vi "StartUp Sequence Open Loop Rev 1.55.vi"() -> ()   [LabVIEW 2017]
panel:
  out "Requested RPM":i32
  out "Waveform Chart":cluster{i32, i32}(graph)
  in  "Set RPM":string
  out "Pump Value 2":string
  in  "Soft Shut Off":bool
  out "Pump Value 1":string
  in  "Send RPM":bool
  in  "Send Command":bool
  in  "Custom Command":string
  out "Startup Success":bool
  in  "Output File":path
  in  "Shut Off":bool
  out "ECU COM Port Out":refnum<visa-resource-name>
  out "Throttle Position":string
  out "Turbine RPM":string
  out "Turbine Temp":string
  out "Error Out":errorcluster
  in  "Error In":errorcluster
  in  "ECU COM Port":refnum<visa-resource-name>
  out "Turbine State":string
  in  "Strt Sqnc":bool
  # "Note: save to a .csv file"
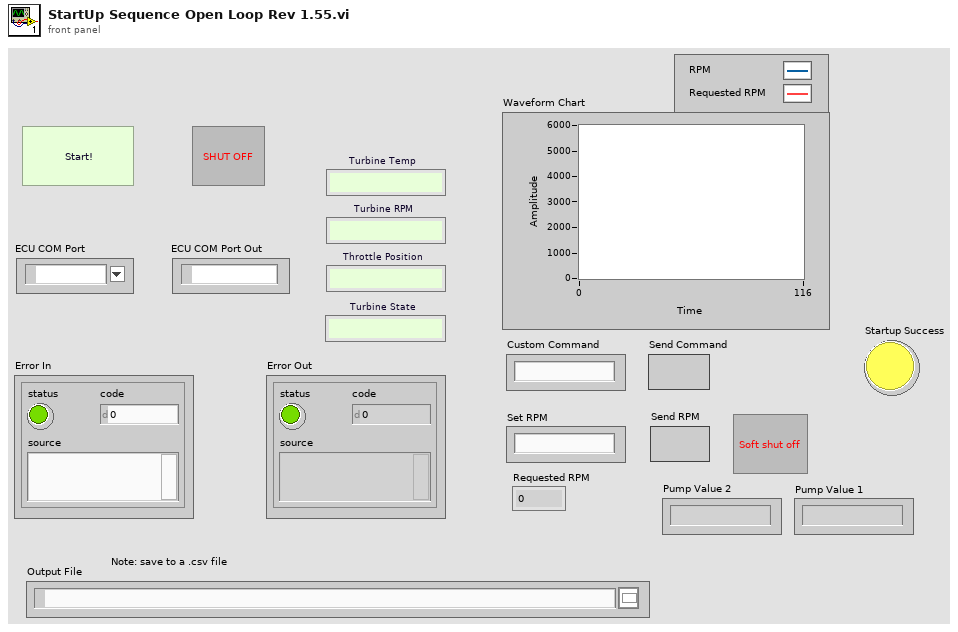
[diagram p1: front panel]
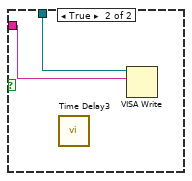
[diagram p3: hidden frame]
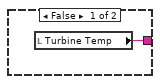
[diagram p4: hidden frame]
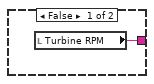
[diagram p5: hidden frame]
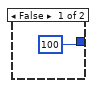
[diagram p7: hidden frame]
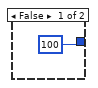
[diagram p8: hidden frame]
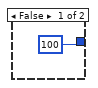
[diagram p9: hidden frame]
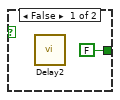
[diagram p11: hidden frame]
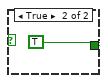
[diagram p12: hidden frame]
diagram:
  w27 = 21 ("Pulse Width")
  w28 = 160 ("Voltage")
  w33 = 16 ("Pulse Width")
  w34 = 160 ("Voltage")
  w24 = 255 ("y")
  w25 = 80 ("y")
  # "Disengage Starter Motor"
  # "Starter Motor 55%"
  # "Start button is inside a while loop that doesn't progess until True"
  # "Fuel Pump Mode 2"
  # "GlowPlugOff"
  # "Start Up\nFuelPumpMode 1"
  # "BurnerValveIgnitionPercent"
  # "If False, each Case structure is set\nto an arbitrary Delay time of 0.2 s"
  # "Each Stage is inside a while loop so that \nthe sequence doesn't progress until True"
  n1 = call "Initialize Com Port.vi"("Error In"="Error In", "ECU COM Port"="ECU COM Port") -> ("Error Out"=w47:errorcluster, "ECU COM Port Out"=w46:refnum<visa-resource-name>)  [unwired: 8 in]
  n2 = while {
    tunnel: w47 -> [w99]
    tunnel: [w99] -> w45
    stop <- "Strt Sqnc" stop-if-true
  }
  n3 = call "Initialize Output File.vi"("error in (no error)"=w45, "File Path Control"="Output File") -> ("error out"=w23:errorcluster)  [unwired: 9 in]
  n4 = flat-sequence {
    tunnel: w23 -> [w101]
    tunnel: [w101] -> w38
    frame #0 {
      n5 = local write "Strt Sqnc"(FALSE ("Strt Sqnc")) -> ()
    }
  }
  n6 = flat-sequence {
    tunnel: [w104] -> w22
    tunnel: w23 -> [w104]
    frame #0 {
      w103 = "0" ("Pump Value 1")
      n7 = local write "Pump Value 2"(w103) -> ()
      n8 = local write "Pump Value 1"(w103) -> ()
    }
  }
  n9 = while {
    tunnel: w22 -> [w131]
    tunnel: w46 -> [w130]
    tunnel: "Output File" -> [w127]
    stop <- w126 continue-if-true
    n10 = call "Get Engine Update.vi"("Error In"=w131, "ECU COM Port"=w130) -> ("Error Out"=w128:errorcluster, "Temperature"=w113:string, "RPMs"=w115:string, "ECU COM Port Out"=w125:refnum<visa-resource-name>)  [unwired: 6 in]
    n11 = call "Time Delay4"() -> ()  [unwired: 11 in, 1 out]
    n12 = Decimal String To Number(string=w115) -> (number=w111:i32)  [unwired: 2 in, 1 out]
    n13 = call "Safety Check.vi"("Temperature"=w113, "RPMs"=w115) -> ("Safe?"=w126:bool)  [unwired: 9 in]
    n14 = Decimal String To Number(string=w113) -> (number=w112:i32)  [unwired: 2 in, 1 out]
    n15 = Not Equal?(x=w115, y="") -> (x != y?=w110:bool)
    n16 = Not Equal?(x=w113, y="") -> (x != y?=w106:bool)
    n17 = Not Equal To 0?(x=w111) -> (x != 0?=w108:bool)
    n18 = Not Equal To 0?(x=w112) -> (x != 0?=w105:bool)
    n19 = And(x=w110, y=w108) -> (x .and. y?=w109:bool)
    n20 = And(x=w106, y=w105) -> (x .and. y?=w107:bool)
    n21 = case shown="False" w126 {
      selector: w126 -> [w136 w138]
      tunnel: w125 -> [w137 _]
      tunnel: [w136 w138] -> w124
      frame False {
        n22 = call "Emergency Shutoff.vi"("ECU COM Port"=w137) -> ()  [unwired: 9 in, 2 out]
      }
      frame True {
      }
    }
    n23 = case shown="True" w109 {
      tunnel: w115 -> [_ w135]
      tunnel: [w134 w135] -> w121
      frame False {
        n24 = local read "Turbine RPM"() -> (w134:string)
      }
      frame True {
        "Turbine RPM" <- w135
      }
    }
    n25 = case shown="True" w107 {
      tunnel: w113 -> [_ w133]
      tunnel: [w132 w133] -> w120
      frame False {
        n26 = local read "Turbine Temp"() -> (w132:string)
      }
      frame True {
        "Turbine Temp" <- w133
      }
    }
    n27 = Not(x=w124) -> (.not. x?=w129:bool)
    n28 = Stop(stop? (T)=w129) -> ()
    n29 = local read "Requested RPM"() -> (w118:i32)
    n30 = local read "Pump Value 2"() -> (w122:string)
    n31 = local read "Pump Value 1"() -> (w123:string)
    n32 = Decimal String To Number(string=w121) -> (number=w119:i32)  [unwired: 2 in, 1 out]
    n33 = Bundle(w119, "Requested RPM"=w118) -> (→"Waveform Chart":cluster{i32, "Requested RPM":i32})  [unwired: 1 in]
    n34 = call "Write Data to Output File.vi"("Pump Value 2"=w122, "Pump Value 1"=w123, "Error In"=w128, "Temperature"=w120, "RPM"=w121, "File Path Control"=w127) -> ()  [unwired: 5 in, 1 out]
  }
  n35 = while {
    tunnel: w46 -> [w140]
    tunnel: w47 -> [_]
    stop <- FALSE stop-if-true
    n36 = case shown="False" "Send Command" {
      tunnel: "Custom Command" -> [_ w144]
      tunnel: w140 -> [_ w143]
      frame False {
      }
      frame True {
        n37 = call "Time Delay3"() -> ()  [unwired: 11 in, 1 out]
        n38 = VISA Write(VISA resource name=w143, write buffer=w144) -> ()  [unwired: 1 in, 3 out]
      }
    }
  }
  n39 = flat-sequence {
    tunnel: w38 -> [_]
    frame #0 {
      n40 = local write "Turbine State"("Initializing Motor") -> ()
    }
  }
  n41 = while {
    tunnel: ["Shut Off"] -> w96
    tunnel: "ECU COM Port" -> [w146]
    stop <- "Shut Off" stop-if-true
    # "Turns off each individual component"
    n42 = case shown="True" "Shut Off" {
      tunnel: w146 -> [_ w150]
      frame False {
      }
      frame True {
        n43 = call "Emergency Shutoff.vi"("ECU COM Port"=w150) -> ("Error Out"=w149:errorcluster)  [unwired: 9 in, 1 out]
        n44 = local write "Output File"(path "" ("Output File")) -> ()
        n45 = flat-sequence {
          tunnel: w149 -> [w151]
          tunnel: [w151] -> _
          frame #0 {
            n46 = local write "Strt Sqnc"(FALSE ("Strt Sqnc")) -> ()
          }
        }
      }
    }
  }
  n47 = call "Set Glow Plug Duty Cycle.vi"("Error In"=w38, "Duty Cycle"=6, "ECU COM Port"=w46) -> ("Error Out"=w89:errorcluster, "ECU COM Port Out"=w86:refnum<visa-resource-name>)  [unwired: 7 in]
  n48 = call "Delay"("error in (no error)"=w89) -> ("error out"=w88:errorcluster)  [unwired: 10 in]
  n49 = call "Set Glow Plug Duty Cycle.vi"("Error In"=w88, "Duty Cycle"=19, "ECU COM Port"=w86) -> ("Error Out"=w87:errorcluster, "ECU COM Port Out"=w82:refnum<visa-resource-name>)  [unwired: 7 in]
  n50 = call "Delay"("error in (no error)"=w87) -> ("error out"=w83:errorcluster)  [unwired: 10 in]
  n51 = call "Set Starter Motor Duty Cycle.vi"("Error In"=w83, "Duty Cycle"=6, "ECU COM Port"=w82) -> ("Error Out"=w81:errorcluster, "ECU COM Port Out"=w79:refnum<visa-resource-name>)  [unwired: 7 in]
  n52 = call "Set Glow Plug Duty Cycle.vi"("Error In"=w81, "Duty Cycle"=15, "ECU COM Port"=w79) -> ("Error Out"=w80:errorcluster, "ECU COM Port Out"=w75:refnum<visa-resource-name>)  [unwired: 7 in]
  n53 = call "Delay"("error in (no error)"=w80) -> ("error out"=w77:errorcluster)  [unwired: 10 in]
  n54 = call "Set Starter Motor Duty Cycle.vi"("Error In"=w77, "Duty Cycle"=4, "ECU COM Port"=w75) -> ("Error Out"=w76:errorcluster, "ECU COM Port Out"=w74:refnum<visa-resource-name>)  [unwired: 7 in]
  n55 = call "Delay"("error in (no error)"=w76) -> ("error out"=w97:errorcluster)  [unwired: 10 in]
  n56 = Stop(stop? (T)=w96) -> ()
  n57 = while {
    tunnel: w97 -> [w155]
    tunnel: w74 -> [w154]
    tunnel: [w154] -> w36
    tunnel: [w155] -> w98
    stop <- w158 stop-if-true
    n58 = local read "Turbine RPM"() -> (w153:string)
    n59 = Decimal String To Number(string=w153) -> (number=w157:i32)  [unwired: 2 in, 1 out]
    n60 = Greater Or Equal?(x=w157, y=3300) -> (x >= y?=w159:bool)
    n61 = case shown="True" w159 {
      tunnel: [FALSE TRUE] -> w158
      frame False {
        n62 = call "Delay2"() -> ()  [unwired: 11 in, 1 out]
      }
      frame True {
      }
    }
  }
  n63 = flat-sequence {
    tunnel: w97 -> [_]
    frame #0 {
      n64 = local write "Turbine State"("Stage1 Check RPM") -> ()
    }
  }
  n65 = call "CmdSeparator7"("error in (no error)"=w98) -> ("error out"=w32:errorcluster)  [unwired: 10 in]
  n66 = call "Set Pump Fow Rate.vi"("Error In"=w32, "Pulse Width"=w33, "Voltage"=w34, "ECU COM Port"=w36) -> ("Error Out"=w37:errorcluster, "ECU COM Port Out"=w35:refnum<visa-resource-name>)  [unwired: 6 in]
  n67 = flat-sequence {
    tunnel: w34 -> [w164]
    tunnel: w33 -> [w163]
    tunnel: w32 -> [_]
    frame #0 {
      n68 = Number To Decimal String(number=w163) -> (decimal integer string=w165:string)  [unwired: 1 in]
      n69 = Number To Decimal String(number=w164) -> (decimal integer string=w166:string)  [unwired: 1 in]
      n70 = local write "Pump Value 2"(w165) -> ()
      n71 = local write "Pump Value 1"(w166) -> ()
    }
  }
  n72 = call "CmdSeparator2"("error in (no error)"=w37) -> ("error out"=w73:errorcluster)  [unwired: 10 in]
  n73 = call "Set Burner Valve Percent.vi"("Error In"=w73, "Percent"=10, "ECU COM Port"=w35) -> ("Error Out"=w3:errorcluster, "ECU COM Port Out"=w1:refnum<visa-resource-name>)  [unwired: 7 in]
  n74 = while {
    tunnel: [w168] -> w4
    tunnel: w3 -> [w168]
    tunnel: [w167] -> w2
    tunnel: w1 -> [w167]
    stop <- w169 stop-if-true
    n75 = local read "Turbine Temp"() -> (w172:string)
    n76 = Decimal String To Number(string=w172) -> (number=w171:i32)  [unwired: 2 in, 1 out]
    n77 = Greater?(x=w171, y=25) -> (0:w169:bool)
  }
  n78 = for {
    N: 8 -> [_]
    shift-right: [w178] -> _
    shift-left: 27 ("Percent") -> [w180]
    tunnel: w2 -> [w177]
    tunnel: w4 -> [w176]
    tunnel: [w174] -> w19
    tunnel: [w173] -> w18
    n79 = Add(x=w180, y=4 ("Percent")) -> (x+y=w178:i32)
    n80 = call "Set Burner Valve Percent.vi"("Error In"=w176, "Percent"=w178, "ECU COM Port"=w177) -> ("Error Out"=w175:errorcluster, "ECU COM Port Out"=w173:refnum<visa-resource-name>)  [unwired: 7 in]
    n81 = call "CmdSeparator4"("error in (no error)"=w175) -> ("error out"=w174:errorcluster)  [unwired: 10 in]
  }
  n82 = flat-sequence {
    tunnel: w19 -> [_]
    frame #0 {
      n83 = local write "Turbine State"("Stage2 Check Temp.") -> ()
    }
  }
  n84 = while {
    tunnel: [w182] -> _
    tunnel: w19 -> [w184]
    tunnel: [w182] -> w16
    tunnel: [w184] -> w17
    tunnel: w18 -> [w182]
    stop <- w187 stop-if-true
    # "Stage2Temp(C)"
    n85 = local read "Turbine Temp"() -> (w183:string)
    n86 = Decimal String To Number(string=w183) -> (number=w185:i32)  [unwired: 2 in, 1 out]
    n87 = Greater Or Equal?(x=w185, y=90) -> (x >= y?=w188:bool)
    n88 = case shown="False" w188 {
      tunnel: [FALSE TRUE] -> w187
      frame False {
        n89 = call "Delay3"() -> ()  [unwired: 11 in, 1 out]
      }
      frame True {
      }
    }
  }
  n90 = call "Set Glow Plug Duty Cycle.vi"("Error In"=w17, "Duty Cycle"=0, "ECU COM Port"=w16) -> ("Error Out"=w68:errorcluster, "ECU COM Port Out"=w29:refnum<visa-resource-name>)  [unwired: 7 in]
  n91 = call "CmdSeparator3"("error in (no error)"=w68) -> ("error out"=w26:errorcluster)  [unwired: 10 in]
  n92 = call "Set Pump Fow Rate.vi"("Error In"=w26, "Pulse Width"=w27, "Voltage"=w28, "ECU COM Port"=w29) -> ("Error Out"=w31:errorcluster, "ECU COM Port Out"=w30:refnum<visa-resource-name>)  [unwired: 6 in]
  n93 = call "Set Burner Valve Percent.vi"("Error In"=w31, "Percent"=80, "ECU COM Port"=w30) -> ("Error Out"=w65:errorcluster, "ECU COM Port Out"=w66:refnum<visa-resource-name>)  [unwired: 7 in]
  n94 = flat-sequence {
    tunnel: w28 -> [w192]
    tunnel: w27 -> [w191]
    tunnel: w26 -> [_]
    frame #0 {
      n95 = Number To Decimal String(number=w191) -> (decimal integer string=w193:string)  [unwired: 1 in]
      n96 = Number To Decimal String(number=w192) -> (decimal integer string=w194:string)  [unwired: 1 in]
      n97 = local write "Pump Value 2"(w193) -> ()
      n98 = local write "Pump Value 1"(w194) -> ()
    }
  }
  n99 = call "CmdSeparator18"("error in (no error)"=w65) -> ("error out"=w64:errorcluster)  [unwired: 10 in]
  n100 = call "Set Fuel Valve Percent.vi"("Error In"=w64, "Percent"=12, "ECU COM Port"=w66) -> ("Error Out"=w63:errorcluster, "ECU COM Port Out"=w67:refnum<visa-resource-name>)  [unwired: 7 in]
  n101 = call "CmdSeparator16"("error in (no error)"=w63) -> ("error out"=w95:errorcluster)  [unwired: 10 in]
  n102 = for {
    N: 4 -> [_]
    tunnel: [w195] -> _
    tunnel: [w209] -> _
    tunnel: w67 -> [w201]
    tunnel: w95 -> [w202]
    shift-right: [w200] -> w59
    shift-left: 12 -> [w206]
    shift-right: [w197] -> _
    shift-left: 80 -> [w203]
    tunnel: [w209] -> w57 mode=indexing
    tunnel: [w195] -> w60 mode=indexing
    n103 = Less?(x=w206, y=100) -> (x < y?=w207:bool)
    n104 = Less?(x=w203, y=100) -> (x < y?=w204:bool)
    n105 = case shown="True" w204 {
      tunnel: w203 -> [_ w213]
      tunnel: [100 w211] -> w197
      frame False {
      }
      frame True {
        n106 = Add(x=w213, y=5) -> (x+y=w211:i32)
      }
    }
    n107 = case shown="True" w207 {
      tunnel: w206 -> [_ w217]
      tunnel: [100 w215] -> w200
      frame False {
      }
      frame True {
        n108 = Add(x=w217, y=6) -> (x+y=w215:i32)
      }
    }
    n109 = call "Set Fuel Valve Percent.vi"("Error In"=w202, "Percent"=w200, "ECU COM Port"=w201) -> ("Error Out"=w199:errorcluster, "ECU COM Port Out"=w196:refnum<visa-resource-name>)  [unwired: 7 in]
    n110 = call "Set Burner Valve Percent.vi"("Error In"=w199, "Percent"=w197, "ECU COM Port"=w196) -> ("Error Out"=w198:errorcluster, "ECU COM Port Out"=w195:refnum<visa-resource-name>)  [unwired: 7 in]
    n111 = call "CmdSeparator17"("error in (no error)"=w198) -> ("error out"=w209:errorcluster)  [unwired: 10 in]
  }
  n112 = flat-sequence {
    tunnel: w57 -> [_]
    frame #0 {
      n113 = local write "Turbine State"("Pump Ramp Up") -> ()
    }
  }
  n114 = for {
    N: 3 -> [_]
    tunnel: [w225] -> w49
    tunnel: [w236] -> w50
    shift-right: [w232] -> _
    shift-left: w59 -> [w233]
    tunnel: w57 -> [w229] mode=indexing
    tunnel: w60 -> [w228] mode=indexing
    shift-right: [w221] -> _
    shift-left: 21 -> [w222]
    w220 = 160 ("y")
    n115 = Less?(x=w233, y=100) -> (x < y?=w234:bool)
    n116 = Add(x=w222, y=1) -> (x+y=w221:i32)
    n117 = case shown="True" w234 {
      tunnel: w233 -> [_ w244]
      tunnel: [100 w242] -> w232
      frame False {
      }
      frame True {
        n118 = Add(x=w244, y=5) -> (x+y=w242:i32)
      }
    }
    n119 = call "Set Fuel Valve Percent.vi"("Error In"=w229, "Percent"=w232, "ECU COM Port"=w228) -> ("Error Out"=w231:errorcluster, "ECU COM Port Out"=w230:refnum<visa-resource-name>)  [unwired: 7 in]
    n120 = call "Set Burner Valve Percent.vi"("Error In"=w231, "Percent"=100 ("y"), "ECU COM Port"=w230) -> ("Error Out"=w219:errorcluster, "ECU COM Port Out"=w226:refnum<visa-resource-name>)  [unwired: 7 in]
    n121 = call "Set Pump Fow Rate.vi"("Error In"=w219, "Pulse Width"=w221, "Voltage"=w220, "ECU COM Port"=w226) -> ("Error Out"=w224:errorcluster, "ECU COM Port Out"=w225:refnum<visa-resource-name>)  [unwired: 6 in]
    n122 = flat-sequence {
      tunnel: w220 -> [w238]
      tunnel: w221 -> [w237]
      tunnel: w219 -> [_]
      frame #0 {
        n123 = Number To Decimal String(number=w237) -> (decimal integer string=w239:string)  [unwired: 1 in]
        n124 = Number To Decimal String(number=w238) -> (decimal integer string=w240:string)  [unwired: 1 in]
        n125 = local write "Pump Value 2"(w239) -> ()
        n126 = local write "Pump Value 1"(w240) -> ()
      }
    }
    n127 = call "CmdSeparator20"("error in (no error)"=w224) -> ("error out"=w236:errorcluster)  [unwired: 10 in]
  }
  n128 = call "Set Starter Motor Duty Cycle.vi"("Error In"=w50, "Duty Cycle"=11, "ECU COM Port"=w49) -> ("Error Out"=w14:errorcluster, "ECU COM Port Out"=w15:refnum<visa-resource-name>)  [unwired: 7 in]
  n129 = flat-sequence {
    tunnel: w14 -> [_]
    frame #0 {
      n130 = local write "Turbine State"("Secondary Pump Ramp Up") -> ()
    }
  }
  n131 = while {
    tunnel: w15 -> [w250]
    tunnel: w14 -> [w249]
    tunnel: [w248] -> w13
    tunnel: [w247] -> w12
    stop <- w253 stop-if-true
    w252 = 160 ("y")
    n132 = local read "Turbine RPM"() -> (w259:string)
    n133 = Decimal String To Number(string=w259) -> (number=w255:i32)  [unwired: 2 in, 1 out]
    n134 = Multiply(x=w255, y=0.0008) -> (x*y=w257:dbl)
    n135 = call "Set Fuel Valve Percent.vi"("Error In"=w249, "Percent"=100 ("y"), "ECU COM Port"=w250) -> ("Error Out"=w264:errorcluster, "ECU COM Port Out"=w263:refnum<visa-resource-name>)  [unwired: 7 in]
    n136 = Add(x=w257, y=10.537) -> (x+y=w251:dbl)
    n137 = call "Set Burner Valve Percent.vi"("Error In"=w264, "Percent"=0 ("y"), "ECU COM Port"=w263) -> ("Error Out"=w260:errorcluster, "ECU COM Port Out"=w261:refnum<visa-resource-name>)  [unwired: 7 in]
    n138 = call "Set Pump Fow Rate.vi"("Error In"=w260, "Pulse Width"=w251, "Voltage"=w252, "ECU COM Port"=w261) -> ("Error Out"=w246:errorcluster, "ECU COM Port Out"=w248:refnum<visa-resource-name>)  [unwired: 6 in]
    n139 = call "CmdSeparator5"("error in (no error)"=w246) -> ("error out"=w247:errorcluster)  [unwired: 10 in]
    n140 = flat-sequence {
      tunnel: w252 -> [w268]
      tunnel: w251 -> [w267]
      tunnel: [w266] -> _
      tunnel: w246 -> [w266]
      frame #0 {
        n141 = Number To Decimal String(number=w267) -> (decimal integer string=w269:string)  [unwired: 1 in]
        n142 = Number To Decimal String(number=w268) -> (decimal integer string=w270:string)  [unwired: 1 in]
        n143 = local write "Pump Value 2"(w269) -> ()
        n144 = local write "Pump Value 1"(w270) -> ()
      }
    }
    n145 = Greater Or Equal?(x=w255, y=40000) -> (x >= y?=w253:bool)
  }
  n146 = call "Set Pump Fow Rate.vi"("Error In"=w12, "Pulse Width"=w24, "Voltage"=w25, "ECU COM Port"=w13) -> ("Error Out"=w56:errorcluster, "ECU COM Port Out"=w55:refnum<visa-resource-name>)  [unwired: 6 in]
  n147 = flat-sequence {
    tunnel: w25 -> [w273]
    tunnel: w24 -> [w272]
    tunnel: [w271] -> _
    tunnel: w12 -> [w271]
    frame #0 {
      n148 = Number To Decimal String(number=w272) -> (decimal integer string=w274:string)  [unwired: 1 in]
      n149 = Number To Decimal String(number=w273) -> (decimal integer string=w275:string)  [unwired: 1 in]
      n150 = local write "Pump Value 2"(w274) -> ()
      n151 = local write "Pump Value 1"(w275) -> ()
    }
  }
  n152 = while {
    tunnel: w56 -> [w277]
    tunnel: w55 -> [w276]
    tunnel: [w277] -> w52
    tunnel: [w276] -> w54
    stop <- w278 stop-if-true
    n153 = local read "Turbine RPM"() -> (w281:string)
    n154 = Decimal String To Number(string=w281) -> (number=w280:i32)  [unwired: 2 in, 1 out]
    n155 = Greater?(x=w280, y=44000) -> (0:w278:bool)
  }
  n156 = flat-sequence {
    tunnel: w52 -> [_]
    frame #0 {
      n157 = local write "Turbine State"("Acheived Idle RPM!") -> ()
    }
  }
  n158 = call "Set Starter Motor Duty Cycle.vi"("Error In"=w52, "Duty Cycle"=0, "ECU COM Port"=w54) -> ("Error Out"=w43:errorcluster, "ECU COM Port Out"=w42:refnum<visa-resource-name>)  [unwired: 7 in]
  n159 = flat-sequence {
    tunnel: w43 -> [_]
    frame #0 {
      "Startup Success" <- TRUE
    }
  }
  n160 = while {
    tunnel: w42 -> [w297]
    tunnel: [w296] -> w40
    tunnel: [w295] -> w41
    tunnel: w43 -> [w294]
    stop <- "Soft Shut Off" stop-if-true
    # "NOTE:\nThere are data entry limits\non this input. These may need\nto be deleted in the future"
    n161 = Decimal String To Number(string="Set RPM") -> (number=w285:i32)  [unwired: 2 in, 1 out]
    n162 = Less?(x=w285, y=135000) -> (x < y?=w291:bool)
    n163 = Greater?(x=w285, y=44000) -> (0:w286:bool)
    n164 = And(x=w286, y=w291) -> (x .and. y?=w289:bool)
    n165 = call "Time Delay"() -> ()  [unwired: 11 in, 1 out]
    n166 = And(x=w289, y="Send RPM") -> (x .and. y?=w287:bool)
    n167 = case shown="True" w287 {
      tunnel: w297 -> [w298 w308]
      tunnel: w294 -> [w299 w307]
      tunnel: [w298 w306] -> w296
      tunnel: [w299 w305] -> w295
      tunnel: w285 -> [_ w300]
      frame False {
      }
      frame True {
        n168 = call "RPM to Fuel Flow.vi"("Requested RPM"=w300) -> ("Fuel Pump Value 1"=w301:i32)  [unwired: 10 in]
        n169 = call "Set Pump Fow Rate.vi"("Error In"=w307, "Pulse Width"=255, "Voltage"=w301, "ECU COM Port"=w308) -> ("Error Out"=w305:errorcluster, "ECU COM Port Out"=w306:refnum<visa-resource-name>)  [unwired: 6 in]
        n170 = Number To Decimal String(number=w301) -> (decimal integer string=→"Pump Value 1":string)  [unwired: 1 in]
        n171 = local write "Pump Value 2"("255" ("Pump Value 2")) -> ()
        "Requested RPM" <- w300
      }
    }
  }
  n172 = call "Emergency Shutoff.vi"("Error In"=w41, "ECU COM Port"=w40) -> ("Error Out"=w39:errorcluster, "ECU COM Port Out"=w10:refnum<visa-resource-name>)  [unwired: 8 in]
  n173 = flat-sequence {
    tunnel: w39 -> [w310]
    tunnel: [w310] -> w11
    frame #0 {
      w309 = "0"
      n174 = local write "Pump Value 1"(w309) -> ()
      n175 = local write "Pump Value 2"(w309) -> ()
    }
  }
  n176 = while {
    tunnel: w11 -> [w316]
    tunnel: w10 -> [w313]
    tunnel: [w311] -> w9
    tunnel: [w312] -> w8
    stop <- w317 stop-if-true
    n177 = while {
      tunnel: [w322] -> w315
      tunnel: w316 -> [w322]
      stop <- w325 stop-if-true
      n178 = local read "Turbine RPM"() -> (w326:string)
      n179 = Decimal String To Number(string=w326) -> (number=w323:i32)  [unwired: 2 in, 1 out]
      n180 = Less?(x=30000, y=w323) -> (x < y?=w325:bool)
    }
    n181 = local read "Turbine Temp"() -> (w320:string)
    n182 = Decimal String To Number(string=w320) -> (number=w319:i32)  [unwired: 2 in, 1 out]
    n183 = flat-sequence {
      tunnel: w311 -> [_]
      frame #0 {
        n184 = local write "Turbine State"("Cooling Down") -> ()
      }
    }
    n185 = call "Set Starter Motor Duty Cycle.vi"("Error In"=w315, "Duty Cycle"=4, "ECU COM Port"=w313) -> ("Error Out"=w311:errorcluster, "ECU COM Port Out"=w312:refnum<visa-resource-name>)  [unwired: 7 in]
    n186 = Greater?(x=w319, y=100) -> (0:w317:bool)
  }
  n187 = flat-sequence {
    tunnel: w5 -> [_]
    frame #0 {
      n188 = local write "Turbine State"("Off") -> ()
    }
  }
  n189 = call "Set Starter Motor Duty Cycle.vi"("Error In"=w9, "Duty Cycle"=0, "ECU COM Port"=w8) -> ("Error Out"=w5:errorcluster, "ECU COM Port Out"=→"ECU COM Port Out":refnum<visa-resource-name>)  [unwired: 7 in]
  "Error Out" <- w5
